vi "Sandbox MB Engine.vi"() -> ()   [LabVIEW 2019, in "MB_ENGINE.lvclass"]
uses:
  MB_ENGINE_class/MB_ENGINE.lvclass
  MB_ENGINE_class/Switch Rule and Polarity.ctl
  MB_ENGINE_class/Engine State.ctl
  MB_ENGINE_class/Limits Status.ctl
  MB_ENGINE_class/Engine Alarms.ctl
  MB_ENGINE_class/Settings.ctl
  MB_ENGINE_class/cmd enum.ctl
  D:/GIT H4000/H4000/src/modbus engine custom/MB_MODULE_class/MB_MODULE.lvclass
  MB_MODULE_class/MB_MODULE.lvclass/MB_MODULE.ctl
  <vilib>/NI/Modbus Library/API/Wrapper/Create TCP Master.vi
  <vilib>/NI/Modbus Library/API/Wrapper/API Main.lvlib
  MB_MODULE_class/MB_MODULE.lvclass
panel:
  out "Connected":bool
  in  "percent force":u16
  out "Numeric":i32
  in  "Settings W":T1={"ACC Steps Per Sec^2"=16, "DEC Steps Per Sec^2"=16, "Min Velosity Step Per Sec"=0, "Max Velosity Step Per Sec"=16, "MicroStep"=4}
  in  "write setting":bool
  in  "Switch Rule and Polarity  W":T2
  in  "write sw":bool
  in  "stop":bool
  out "error out":errorcluster
  in  "write arg":bool
  in  "write cmd":bool
  in  "ARG U32":i32
  in  "cmd to write":T3 items=["0 Idle"=0, "1 GoTo Absolute Position"=1, "2 GoTo Relative"=2, "10 GoTo Home Position"=10, "11 Set Home Position"=11, "12 Set FindHome Mode"=12, "13 Reset FindHome Mode"=13, "14 Get FindHome State"=14, "20 Hard Stop"=20, "21 HiZ Stop"=21, "22 Soft Stop"=22, "30 Clear Fault"=30, "40 Encoder Set Home"=40, "70 Driver Init"=70]
  out "Settings R":T1
  out "Counter":u16
  out "angle":dbl
  out "Raw":u16
  out "Alarms":T4
  out "Limits":T5
  out "Engine State":T6 items=["ACCELERATING", "DECELERATINGTOSTOP", "DECELERATING", "STEADY", "INDEX_ACCEL", "NDEX_RUN", "INDEX_DECEL", "INDEX_DWELL", "INACTIVE", "STANDBY", "STANDBYTOINACTIVE"]
  out "Switch Rule and Polarity  R":T2
  in  "SW":u16
  out "RAW Possition":i32
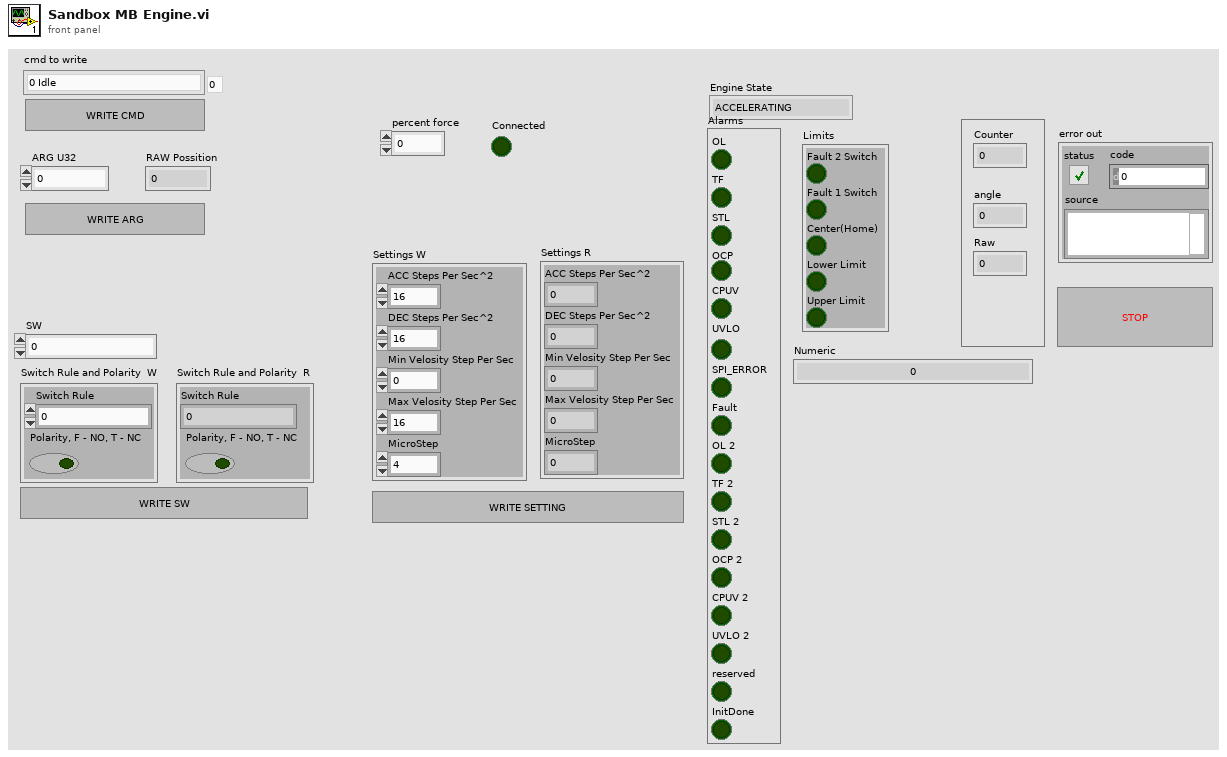
[diagram p1: front panel]
types:
  T1 = typedef "MB_ENGINE.lvclass/Settings.ctl" = cluster{"ACC Steps Per Sec^2":u16, "DEC Steps Per Sec^2":u16, "Min Velosity Step Per Sec":u16, "Max Velosity Step Per Sec":u16, "MicroStep":u16}
  T2 = typedef "MB_ENGINE.lvclass/Switch Rule and Polarity.ctl" = cluster{"Switch Rule":u8, "Polarity, F - NO, T - NC":bool}
  T3 = typedef "MB_ENGINE.lvclass/cmd enum.ctl" = u16
  T4 = typedef "MB_ENGINE.lvclass/Engine Alarms.ctl" = cluster{"OL":bool, "TF":bool, "STL":bool, "OCP":bool, "CPUV":bool, "UVLO":bool, "SPI_ERROR":bool, "Fault":bool, "OL 2":bool, "TF 2":bool, "STL 2":bool, "OCP 2":bool, "CPUV 2":bool, "UVLO 2":bool, "reserved":bool, "InitDone":bool}
  T5 = typedef "MB_ENGINE.lvclass/Limits Status.ctl" = cluster{"Fault 2 Switch":bool, "Fault 1 Switch":bool, "Center(Home)":bool, "Lower Limit":bool, "Upper Limit":bool}
  T6 = typedef "MB_ENGINE.lvclass/Engine State.ctl" = u16
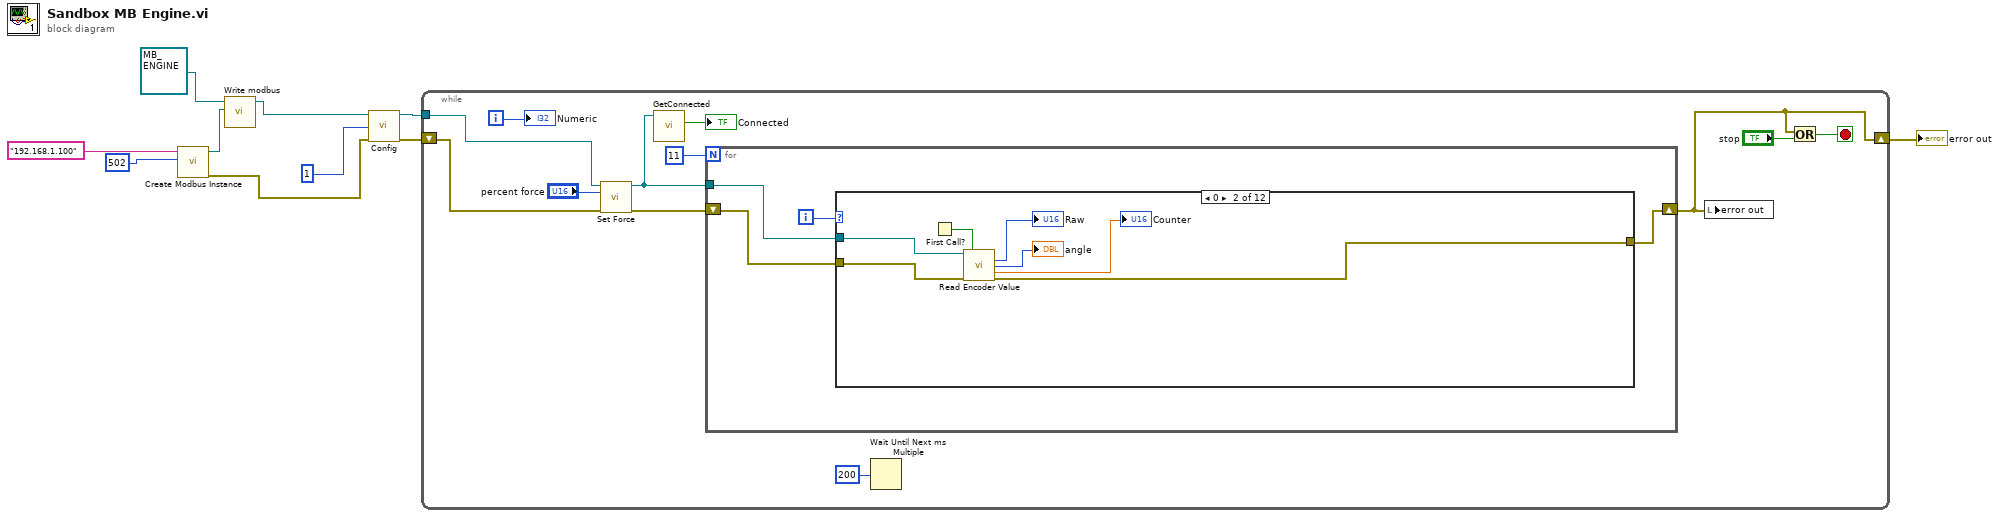
[diagram p0: block diagram]
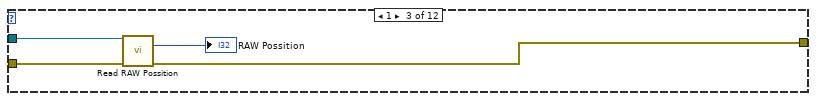
[diagram p3: hidden frame]
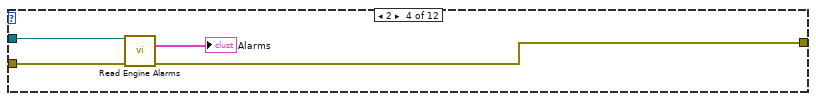
[diagram p4: hidden frame]
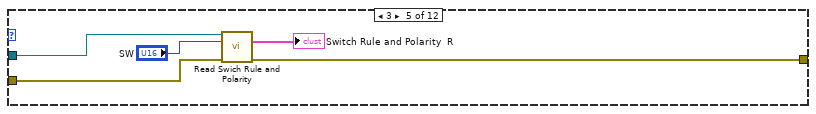
[diagram p5: hidden frame]
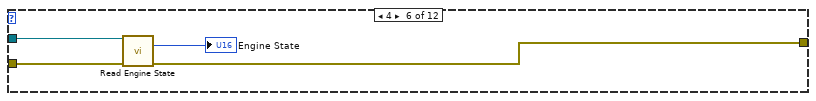
[diagram p6: hidden frame]
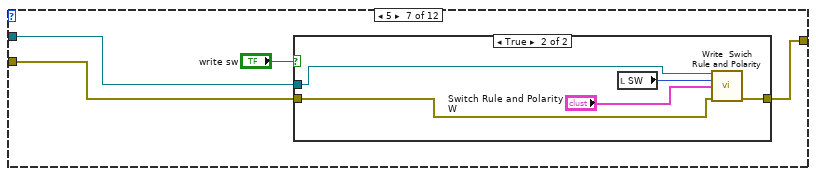
[diagram p7: hidden frame]
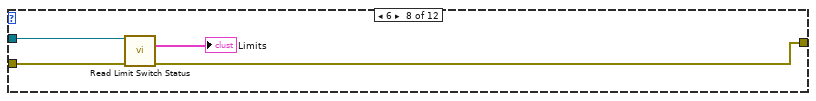
[diagram p9: hidden frame]
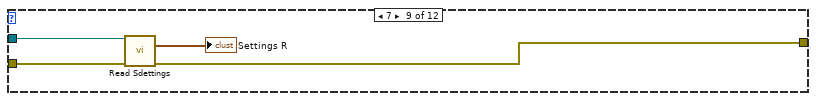
[diagram p10: hidden frame]
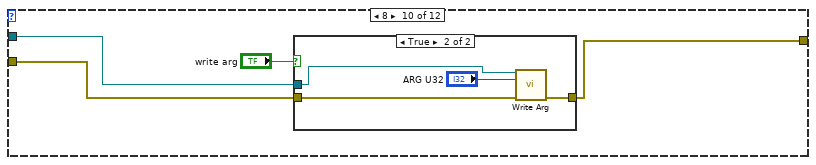
[diagram p11: hidden frame]
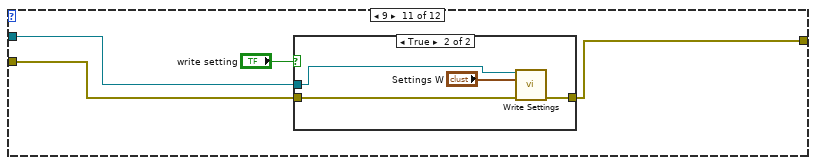
[diagram p13: hidden frame]
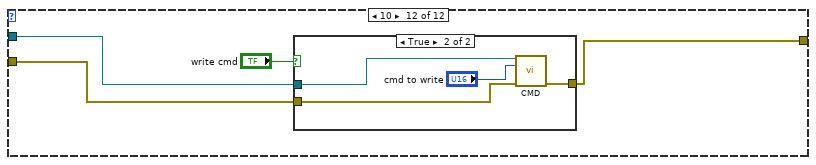
[diagram p15: hidden frame]
diagram:
  n1 = call-poly <vilib>:"Create Modbus Instance.vi"("port (502)"=u16 502, "address"="192.168.1.100") -> ("error out"=w10:errorcluster, "TCP master instance"=w2:refnum<class "Modbus Master.lvclass">)  [unwired: 8 in]
  n2 = call "Write modbus.vi"("Modbus Master"=w2, "MB_MODULE in"=refnum<class "MB_ENGINE.lvclass"> refnum ("class data in")) -> ("MB_MODULE out"=w1:refnum<class "MB_ENGINE.lvclass">)  [unwired: 9 in]
  n3 = call-dynamic "Config.vi"("class data in"=w1, "addres"=u16 1 ("module index"), "error in (no error)"=w10) -> ("class data out"=w8:refnum<class "MB_ENGINE.lvclass">, "error out"=w7:errorcluster)  [unwired: 11 in]
  n4 = while {
    tunnel: w8 -> [w16]
    shift-right: [w18] -> w6
    shift-left: w7 -> [w14]
    i -> [w17]
    stop <- w20 stop-if-true
    n5 = call "Set Force.vi"("class data in"=w16, "percent"="percent force", "error in (no error)"=w14) -> ("class data out"=w12:refnum<class "MB_ENGINE.lvclass">, "error out"=w13:errorcluster)  [unwired: 11 in]
    n6 = call "GetConnected.vi"("MB_MODULE in"=w12) -> ("Connected"=→"Connected":bool)  [unwired: 10 in]
    n7 = for {
      N: 11 -> [_]
      tunnel: w12 -> [w25]
      shift-right: [w24] -> w18
      shift-left: w13 -> [w26]
      i -> [w23]
      n8 = case shown="0" w23 {
        tunnel: w26 -> [w27 w31 w36 w40 w45 w49 w54 w63 w67 w71 w80 w89]
        tunnel: w25 -> [_ w30 w37 w41 w46 w50 w53 w64 w68 w72 w81 w90]
        tunnel: [w27 w29 w35 w39 w43 w48 w52 w62 w66 w70 w79 w88] -> w24
        frame Default {
        }
        frame 0 {
          n9 = First Call?() -> (First Call?: T/F=w28:bool)
          n10 = call "Read Encoder Value.vi"("class data in"=w30, "init"=w28, "error in (no error)"=w31) -> ("type"=→"Raw":u16, "Encoder"=→"angle":i32, "Angel (rad)"=→"Counter":dbl, "error out"=w29:errorcluster)  [unwired: 8 in, 1 out]
        }
        frame 1 {
          n11 = call "Read RAW Possition.vi"("class data in"=w37, "error in (no error)"=w36) -> ("RAW Possition"=→"RAW Possition":i32, "error out"=w35:errorcluster)  [unwired: 11 in, 1 out]
        }
        frame 2 {
          n12 = call "Read Engine Alarms.vi"("class data in"=w41, "error in (no error)"=w40) -> ("Alarms"=→"Alarms":T4, "error out"=w39:errorcluster)  [unwired: 11 in, 1 out]
        }
        frame 3 {
          n13 = call-dynamic "Read Swich Rule and Polarity.vi"("class data in"=w46, "SW"="SW", "error in (no error)"=w45) -> ("Switch Rule and Polarity"=→"Switch Rule and Polarity  R":T2, "error out"=w43:errorcluster)  [unwired: 10 in, 1 out]
        }
        frame 4 {
          n14 = call "Read Engine State.vi"("class data in"=w50, "error in (no error)"=w49) -> ("Engine State"=→"Engine State":T6, "error out"=w48:errorcluster)  [unwired: 11 in, 1 out]
        }
        frame 5 {
          n15 = case shown="True" "write sw" {
            tunnel: [w56 w61] -> w52
            tunnel: w54 -> [w56 w58]
            tunnel: w53 -> [_ w57]
            frame False {
            }
            frame True {
              n16 = local read "SW"() -> (w59:u16)
              n17 = call-dynamic "Write  Swich Rule and Polarity.vi"("class data in"=w57, "SW"=w59, "Switch Rule and Polarity"="Switch Rule and Polarity  W", "error in (no error)"=w58) -> ("error out"=w61:errorcluster)  [unwired: 10 in, 1 out]
            }
          }
        }
        frame 6 {
          n18 = call "Read Limit Switch Status.vi"("class data in"=w64, "error in (no error)"=w63) -> ("Limits"=→"Limits":T5, "error out"=w62:errorcluster)  [unwired: 11 in, 1 out]
        }
        frame 7 {
          n19 = call "Read Sdettings.vi"("class data in"=w68, "error in (no error)"=w67) -> ("cluster"=→"Settings R":T1, "error out"=w66:errorcluster)  [unwired: 11 in, 1 out]
        }
        frame 8 {
          n20 = case shown="True" "write arg" {
            tunnel: [w74 w77] -> w70
            tunnel: w72 -> [_ w76]
            tunnel: w71 -> [w74 w75]
            frame False {
            }
            frame True {
              n21 = call "Write Arg.vi"("class data in"=w76, "ARG U32"="ARG U32", "error in (no error)"=w75) -> ("error out"=w77:errorcluster)  [unwired: 11 in, 1 out]
            }
          }
        }
        frame 9 {
          n22 = case shown="True" "write setting" {
            tunnel: [w83 w87] -> w79
            tunnel: w81 -> [_ w85]
            tunnel: w80 -> [w83 w84]
            frame False {
            }
            frame True {
              n23 = call "Write Settings.vi"("class data in"=w85, "cluster"="Settings W", "error in (no error)"=w84) -> ("error out"=w87:errorcluster)  [unwired: 11 in, 1 out]
            }
          }
        }
        frame 10 {
          n24 = case shown="True" "write cmd" {
            tunnel: [w92 w95] -> w88
            tunnel: w90 -> [_ w94]
            tunnel: w89 -> [w92 w93]
            frame False {
            }
            frame True {
              n25 = call "CMD.vi"("class data in"=w94, "cmd to write"="cmd to write", "error in (no error)"=w93) -> ("error out"=w95:errorcluster)  [unwired: 11 in, 1 out]
            }
          }
        }
      }
    }
    n26 = Wait Until Next ms Multiple(millisecond multiple=u32 200) -> ()  [unwired: 1 out]
    n27 = local write "error out"(w18) -> ()
    n28 = Or(x=w18, y="stop") -> (x .or. y?=w20:bool)
    "Numeric" <- w17
  }
  "error out" <- w6
